vi "disable_enable_buttons.vi"(0 "Disabled":T1(ring), 1 "Interrupt":refnum<vi>, 2 "Save Specs":refnum<vi>, 3 "Validate":refnum<vi>, 4 "Bool 1":refnum<vi>, 5 "Bool 2":refnum<vi>, 6 "Bool 3":refnum<vi>, 7 "Bool 9":refnum<vi>, 8 "Bool 4":refnum<vi>, 9 "Bool 8":refnum<vi>, 10 "Bool 5":refnum<vi>, 11 "Bool 7":refnum<vi>, 12 "Bool 6":refnum<vi>) -> ()   [LabVIEW 2019]
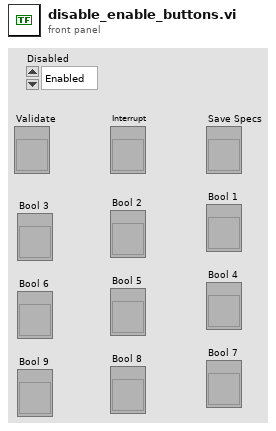
[diagram p1: front panel]
types:
  T1 = enum8{"Enabled", "Disabled", "Disabled and Grayed Out"}
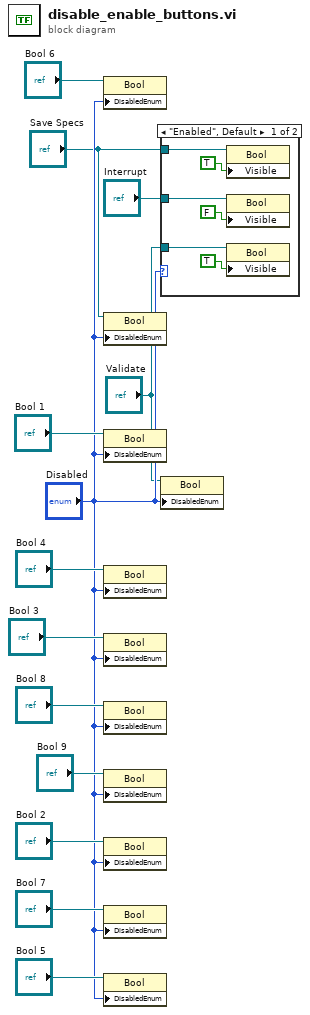
[diagram p0: block diagram]
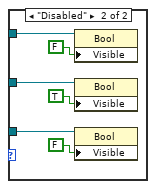
[diagram p2: hidden frame]
diagram:
  n1 = property on="Property Node" class="Bool"(reference="Bool 6", "DisabledEnum"="Disabled") -> ()  [unwired: 1 in, 2 out]
  n2 = property on="Property Node" class="Bool"(reference="Save Specs", "DisabledEnum"="Disabled") -> ()  [unwired: 1 in, 2 out]
  n3 = property on="Property Node" class="Bool"(reference="Bool 1", "DisabledEnum"="Disabled") -> ()  [unwired: 1 in, 2 out]
  n4 = property on="Property Node" class="Bool"(reference="Bool 4", "DisabledEnum"="Disabled") -> ()  [unwired: 1 in, 2 out]
  n5 = property on="Property Node" class="Bool"(reference="Bool 3", "DisabledEnum"="Disabled") -> ()  [unwired: 1 in, 2 out]
  n6 = property on="Property Node" class="Bool"(reference="Bool 8", "DisabledEnum"="Disabled") -> ()  [unwired: 1 in, 2 out]
  n7 = property on="Property Node" class="Bool"(reference="Bool 9", "DisabledEnum"="Disabled") -> ()  [unwired: 1 in, 2 out]
  n8 = property on="Property Node" class="Bool"(reference="Bool 2", "DisabledEnum"="Disabled") -> ()  [unwired: 1 in, 2 out]
  n9 = property on="Property Node" class="Bool"(reference="Bool 7", "DisabledEnum"="Disabled") -> ()  [unwired: 1 in, 2 out]
  n10 = property on="Property Node" class="Bool"(reference="Bool 5", "DisabledEnum"="Disabled") -> ()  [unwired: 1 in, 2 out]
  n11 = case shown="\"Enabled\", Default" "Disabled" {
    tunnel: "Interrupt" -> [w19 w25]
    tunnel: "Validate" -> [w15 w23]
    tunnel: "Save Specs" -> [w14 w21]
    frame "Enabled", Default {
      n12 = property class="Bool"(reference=w14, "Visible"=TRUE) -> ()  [unwired: 1 in, 2 out]
      n13 = property class="Bool"(reference=w19, "Visible"=FALSE) -> ()  [unwired: 1 in, 2 out]
      n14 = property class="Bool"(reference=w15, "Visible"=TRUE) -> ()  [unwired: 1 in, 2 out]
    }
    frame "Disabled" {
      n15 = property class="Bool"(reference=w21, "Visible"=FALSE) -> ()  [unwired: 1 in, 2 out]
      n16 = property class="Bool"(reference=w25, "Visible"=TRUE) -> ()  [unwired: 1 in, 2 out]
      n17 = property class="Bool"(reference=w23, "Visible"=FALSE) -> ()  [unwired: 1 in, 2 out]
    }
  }
  n18 = property on="Property Node" class="Bool"(reference="Validate", "DisabledEnum"="Disabled") -> ()  [unwired: 1 in, 2 out]
